vi "Create new sequence.vi"(7 "Sequence name":string, 11 "error in (no error)":errorcluster) -> (15 "error out":errorcluster)   [LabVIEW 2011]
uses:
  Sequence steps config..ctl
  Single criteria cluster.ctl
  Criteria types.ctl
  Boolean operation.ctl
  <vilib>/Utility/libraryn.llb/Check if File or Folder Exists.vi
  <vilib>/Utility/config.llb/NI_LVConfig.lvlib
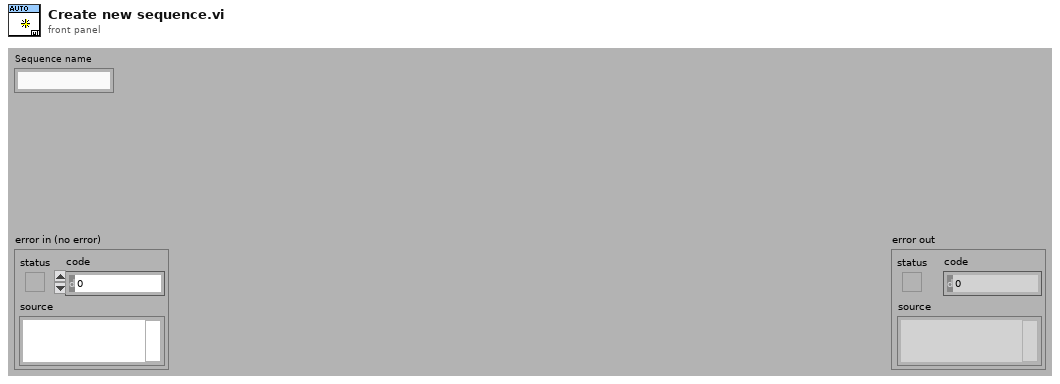
[diagram p1: front panel]
types:
  T1 = typedef "Sequence steps config..ctl" = cluster{"Enabled":bool, "Criteria 1":T2, "C1 op C2":T4, "Criteria 2":T2, "Action index":i32, "Action Name":string, "Action value":dbl}
  T2 = typedef "Single criteria cluster.ctl" = cluster{"Criteria":T3, "Time or analog value":dbl, "Primary IO index":i32, "Secondary  IO index":i32, "User_input":bool}
  T3 = typedef "Criteria types.ctl" = enum16{"No criteria(True)", "Time(s)", "Analog IO over", "Analog IO over or equal", "Analog IO under", "Analog IO under or equal", "Analog IO 1 minus Analog IO 2 over", "Digital IO True", "Digital IO False", "Operator approval"}
  T4 = typedef "Boolean operation.ctl" = enum16{"And", "Or", "Xor", "Nand", "Nor", "Nxor", "Implies"}
  T5 = typedef "NI_LVConfig.lvlib/Config Data RefNum.ctl" = refnum<k1>
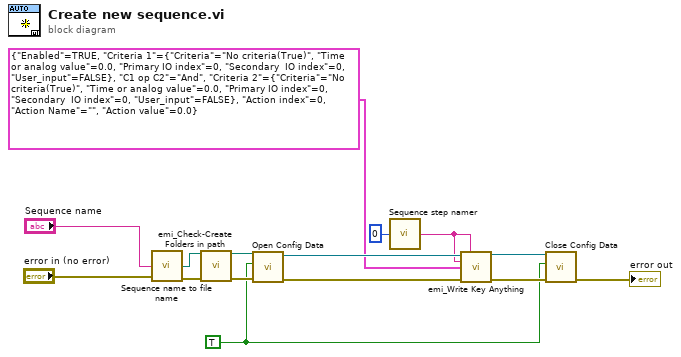
[diagram p0: block diagram]
diagram:
  w1 = TRUE ("create file if necessary (T)")
  n1 = call "Sequence name to file name.vi"("Sequence name"="Sequence name", "error in (no error)"="error in (no error)") -> ("Sequence file path"=w13:path, "error out"=w12:errorcluster)  [unwired: 12 in]
  n2 = call "emi_Check-Create Folders in path.vi"("Path including file"=w13, "error in (no error)"=w12) -> ("Path out"=w9:path, "error out"=w10:errorcluster)  [unwired: 11 in, 1 out]
  n3 = call <vilib>:"Open Config Data.vi"("error in (no error)"=w10, "create file if necessary (T)"=w1, "configuration file path"=w9) -> ("error out"=w5:errorcluster, "refnum"=w11:T5)  [unwired: 6 in, 1 out]
  n4 = call "Sequence step namer.vi"("number"=0) -> ("Step name"=w7:string)
  n5 = call "emi_Write Key Anything.vi"("Ini file refnum"=w11, "Section(Default)"=w7, "Name"=w7, "Anything"=T1 {"Enabled"=TRUE, "Criteria 1"={"Criteria"=enum."No criteria(True)", "Time or analog value"=0.0, "Primary IO index"=0, "Secondary  IO index"=0, "User_input"=FALSE}, "C1 op C2"=enum."And", "Criteria 2"={"Criteria"=enum."No criteria(True)", "Time or analog value"=0.0, "Primary IO index"=0, "Secondary  IO index"=0, "User_input"=FALSE}, "Action index"=0, "Action Name"="", "Action value"=0.0} ("data step cluster"), "error in (no error)"=w5) -> ("Ini file refnum out"=w2:T5, "error out"=w3:errorcluster)  [unwired: 9 in]
  n6 = call <vilib>:"Close Config Data.vi"("error in (no error)"=w3, "write file if changed (T)"=w1, "refnum"=w2) -> ("error out"=→"error out":errorcluster)  [unwired: 7 in, 1 out]
